vi "Opdracht_1.vi"() -> ()   [LabVIEW 2018]
uses:
  <vilib>/Analysis/2dsp.llb/Real FFT.vi
  <vilib>/Analysis/NI_AALPro.lvlib
panel:
  in  "stop":bool
  out "XY Graph 3":cluster{dbl[], sgl[]}(graph)
  in  "Lin (0)/ Log (1)":u8
  out "XY Graph 2":cluster{sgl[], dbl[]}(graph)
  in  "fs":sgl
  in  "file (use dialog)":path
  out "Raw Data":string
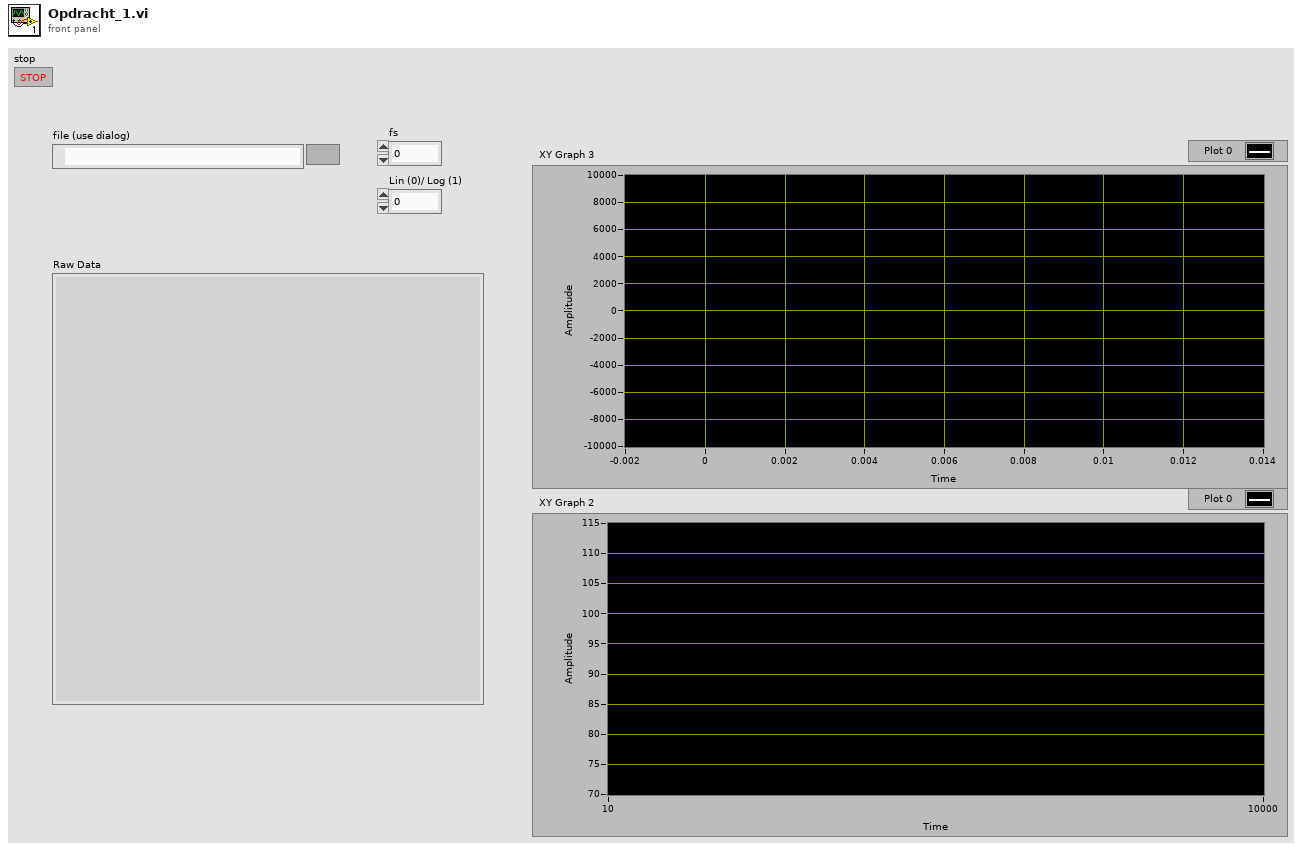
[diagram p1: front panel]
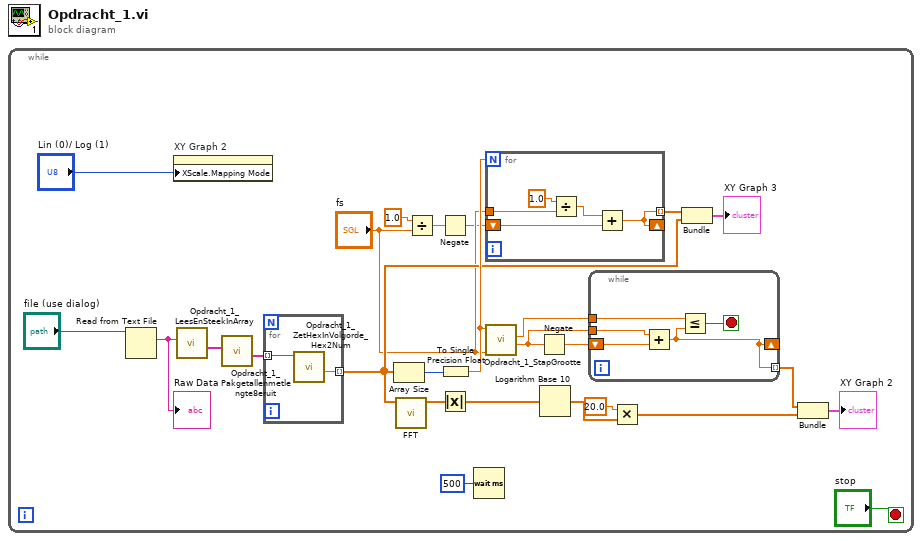
[diagram p0: block diagram]
diagram:
  n1 = while {
    stop <- "stop" stop-if-true
    n2 = Read from Text File(file (use dialog)="file (use dialog)") -> (text=w25:string)  [unwired: 3 in, 3 out]
    "Raw Data" <- w25
    n3 = property on="XY Graph 2" class="XYGraph (strict)"("XScale.Mapping Mode"="Lin (0)/ Log (1)") -> ()  [unwired: 2 in, 2 out]
    n4 = call "Opdracht_1_LeesEnSteekInArray.vi"("String 2"=w25) -> ("array w/ subset deleted"=w20:string[])  [unwired: 10 in]
    n5 = call "Opdracht_1_Pakgetallenmetlengte8eruit.vi"("array w/ subset deleted"=w20) -> ("Array"=w12:string[])  [unwired: 9 in, 1 out]
    n6 = for {
      tunnel: [w37] -> w8 mode=indexing
      tunnel: w12 -> [w38] mode=indexing
      n7 = call "Opdracht_1_ZetHexInVolgorde_Hex2Num.vi"("Getallen"=w38) -> ("*(type *) &x"=w37:sgl)  [unwired: 10 in]
    }
    n8 = Array Size(array=w8) -> (size(s)=w21:i32)
    n9 = call-poly <vilib>:"FFT.vi"("X"=w8) -> ("FFT {X}"=w13:cdb[])  [unwired: 9 in, 1 out]
    n10 = Divide(x=sgl 1.0, y="fs") -> (x/y=w4:sgl)
    n11 = Negate(x=w4) -> (-x=w3:sgl)
    n12 = Absolute Value(x=w13) -> (abs(x)=w14:dbl[])
    n13 = To Single Precision Float(number=w21) -> (single precision float=w10:sgl)
    n14 = Wait (ms)(milliseconds to wait=u32 500) -> ()  [unwired: 1 out]
    n15 = for {
      N: w10 -> [_]
      tunnel: "fs" -> [w30]
      shift-right: [w27] -> _
      shift-left: w3 -> [w28]
      tunnel: [w27] -> w7 mode=indexing
      n16 = Divide(x=1.0, y=w30) -> (x/y=w29:dbl)
      n17 = Add(x=w29, y=w28) -> (x+y=w27:dbl)
    }
    n18 = call "Opdracht_1_StapGrootte.vi"("fs"="fs", "N"=w10) -> ("Stapgrootte"=w22:sgl, 2:w24:sgl)  [unwired: 8 in]
    n19 = Negate(x=w22) -> (-x=w23:sgl)
    n20 = Logarithm Base 10(1:w14) -> (0:w19:dbl[])
    n21 = while {
      shift-right: [w32] -> _
      shift-left: w23 -> [w36]
      tunnel: w22 -> [w35]
      tunnel: w24 -> [w34]
      tunnel: [w32] -> w15 mode=indexing
      stop <- w33 stop-if-true
      n22 = Add(x=w35, y=w36) -> (x+y=w32:sgl)
      n23 = Less Or Equal?(x=w34, y=w32) -> (x <= y?=w33:bool)
    }
    n24 = Multiply(x=20.0, y=w19) -> (x*y=w16:dbl[])
    n25 = Bundle(w7, w8) -> (→"XY Graph 3":cluster{dbl[], sgl[]})  [unwired: 1 in]
    n26 = Bundle(w15, w16) -> (→"XY Graph 2":cluster{sgl[], dbl[]})  [unwired: 1 in]
  }
